vi "Temp and humidity.vi"() -> ()   [LabVIEW 2018]
uses:
  <vilib>/Instr/_visa.llb/VISA Configure Serial Port (Instr).vi
panel:
  out "Humidity":dbl(graph)
  out "Temperature":dbl(graph)
  in  "stop":bool
  out "Temperature":dbl
  out "Humidity":dbl
  in  "VISA resource name":refnum<visa-resource-name>="COM4"
  # "Temperature and Humidity sensor"
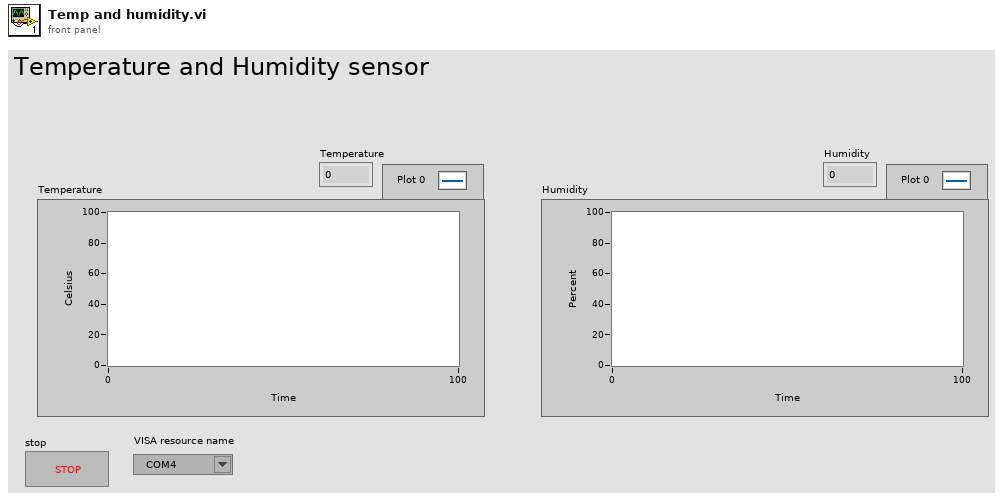
[diagram p1: front panel]
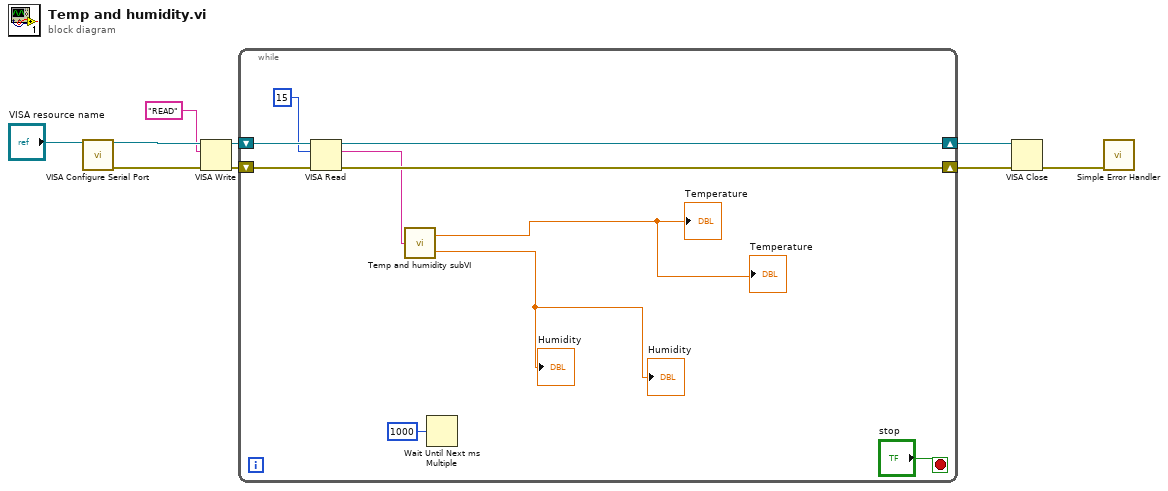
[diagram p0: block diagram]
diagram:
  n1 = call-poly "VISA Configure Serial Port"("VISA resource name"="VISA resource name") -> ("VISA resource name out"=w8:refnum<visa-resource-name>, "error out"=w5:errorcluster)  [unwired: 13 in]
  n2 = VISA Write(VISA resource name=w8, write buffer="READ", error in (no error)=w5) -> (VISA resource name out=w7:refnum<visa-resource-name>, error out=w4:errorcluster)  [unwired: 1 out]
  n3 = while {
    shift-right: [w18] -> w6
    shift-left: w7 -> [w19]
    shift-right: [w16] -> w3
    shift-left: w4 -> [w17]
    stop <- "stop" stop-if-true
    n4 = VISA Read(VISA resource name=w19, byte count=u32 15, error in (no error)=w17) -> (VISA resource name out=w18:refnum<visa-resource-name>, read buffer=w12:string, error out=w16:errorcluster)  [unwired: 1 out]
    n5 = call "Temp and humidity subVI.vi"("String"=w12) -> ("Temperature"=→"Temperature" →"Temperature":dbl, "Humidity"=→"Humidity" →"Humidity":dbl)
    n6 = Wait Until Next ms Multiple(millisecond multiple=u32 1000) -> ()  [unwired: 1 out]
  }
  n7 = VISA Close(VISA resource name=w6, error in (no error)=w3) -> (error out=w2:errorcluster)
  n8 = call <vilib>:"Simple Error Handler.vi"("error in (no error)"=w2) -> ()  [unwired: 4 in, 5 out]
